vi "STEP SPEED SEQUENCE.vi"(8 "error in (no error)":errorcluster, 11 "main ref":T1) -> (0 "error out":errorcluster)   [LabVIEW 2025]
uses:
  controls/LAB-IQ UI Data.ctl
  Traction Loop/Traction Receipe Enum.ctl
  STEP SPEED SEQUENCE ENUM.ctl
  SWAY vi's/Sway Write enum.ctl
  LOAD CELL CODE/STEP LOAD SEQUENCE ENUM.ctl
panel:
  in  "Checkbox":bool
  out "ELAPSED TIMER":dbl
  out "Test Size":i32
  in  "Time Index":i32
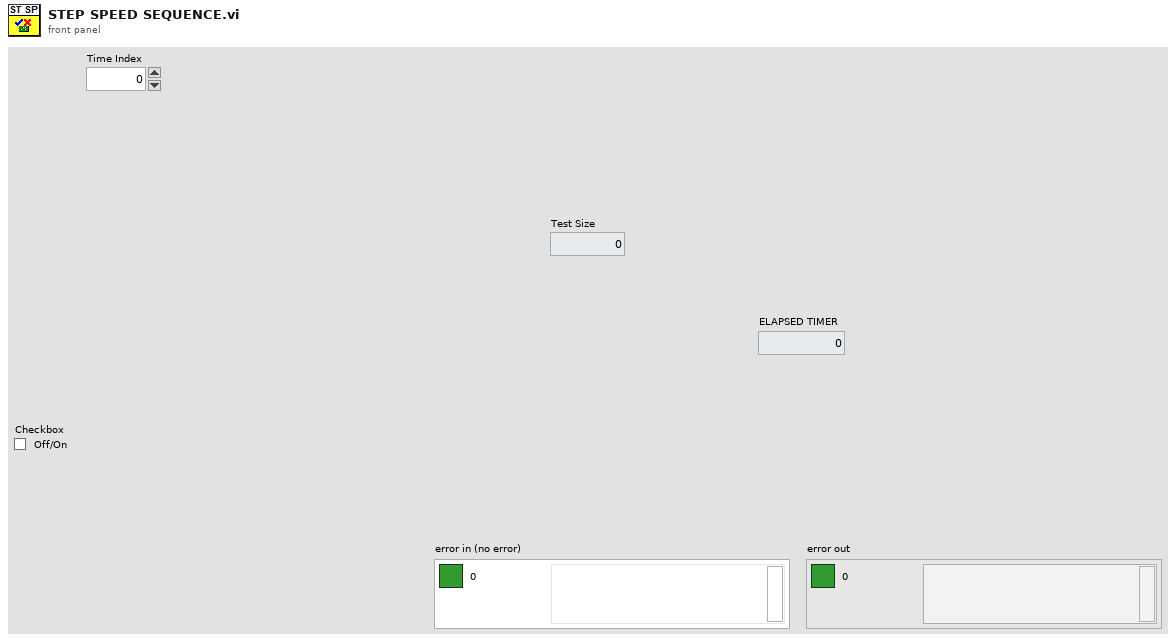
[diagram p1: front panel]
types:
  T1 = typedef "LAB-IQ UI Data.ctl" = cluster{"Main Home Screen":cluster{"GUI":refnum<vi>, "Platform Settings":refnum<vi>, "Configure":refnum<vi>, "Home":refnum<vi>, "EXIT":refnum<vi>, "service 2":refnum<vi>, "MainPage":refnum<vi>, "Analysis":refnum<vi>}, "Platform Settings":cluster{"mm/s  Surge":refnum<vi>, "Drive Error":refnum<vi>, "Disable Axis Jog Soft Limits":refnum<vi>, "mm/s  Sway":refnum<vi>, "Sway and Surge COM Status":refnum<vi>, "Heave COM Status":refnum<vi>, "Enable Platform":refnum<vi>, "Surge Forward Main":refnum<vi>, "Sway Right Main":refnum<vi>, "Sway Left Main":refnum<vi>, "Heave Down Main":refnum<vi>, "Heave Up main":refnum<vi>, "mm/s Heave":refnum<vi>, "mm/sec":refnum<vi>, "mm":refnum<vi>, "Surge Backward Main":refnum<vi>}, "Analysis Screen":cluster{"Analysis Home":refnum<vi>, "Surface Analysis":refnum<vi>, "Imaging":refnum<vi>, "Image Analysis":refnum<vi>, "Post Analysis":refnum<vi>}, "Config Screen":cluster{"Select Load Head":refnum<vi>, "Notes :":refnum<vi>, "FILE":refnum<vi>, "Sample ID :":refnum<vi>, "Operator ID :":refnum<vi>, "Operator Name :":refnum<vi>, "Auto":refnum<vi>}, "Motion Module":cluster{"zNL":refnum<vi>, "NL disp":refnum<vi>, "Rotary Tab":refnum<vi>, "Motion Direction:  3":refnum<vi>, "E.Velocity 2":refnum<vi>, "e.v/ssr 2":refnum<vi>, "Enter Fixed E.Velocity 2":refnum<vi>, "Enter Final SRR 2":refnum<vi>, "Enter initial SRR 2":refnum<vi>, "Enter Fixed SRR 2":refnum<vi>, "Enter the Final E.Velocity (m/s) 2":refnum<vi>, "Enter initial E.Velocity (m/s) 2":refnum<vi>, "Final Speed (RPM) 3":refnum<vi>, "Initial Speed (RPM) 2":refnum<vi>, "Enter the Final Velocity (m/s) 3":refnum<vi>, "Enter initial Velocity (m/s)  3":refnum<vi>, "Ramp Up 2":refnum<vi>, "TEST SELECTION":refnum<vi>, "SPEED SELECTION : ":refnum<vi>, "Angular Oscillation Set":refnum<vi>, "Traction":refnum<vi>, "Step Speed":refnum<vi>, "StepTable For Load-Speed":refnum<vi>, "StepTable For Speed":refnum<vi>, "Surge Forward MM":refnum<vi>, "Surge Backward MM":refnum<vi>, "M3 Image":refnum<vi>, "String 39":refnum<vi>, "Sway Left MM":refnum<vi>, "Sway Right MM":refnum<vi>, "Disable Axis Jog Soft Limits":refnum<vi>, "mm":refnum<vi>, "Heave Down MM":refnum<vi>, "Heave Up MM":refnum<vi>, "Wear Track Diameter (mm)":refnum<vi>, "Set WTD":refnum<vi>, "HomeScratch":refnum<vi>, "HomeRot":refnum<vi>, "PlaceModule":refnum<vi>, "Enter the Angle (Deg)":refnum<vi>, "Enter the Frequency (Hz)":refnum<vi>, "Motion Mode:":refnum<vi>, "LR Sway":refnum<vi>, "Rot Hor":refnum<vi>, "Scratch":refnum<vi>, "LR Cam":refnum<vi>, "MMBack":refnum<vi>, "MMNext":refnum<vi>, "Rot Ver":refnum<vi>, "Rotary Module Selection":refnum<vi>, "calculate rotary":refnum<vi>, "SPEED SELECTION : rotary":refnum<vi>, "Import 2":refnum<vi>, "Save 2":refnum<vi>, "File Path :  2":refnum<vi>, "String 45":refnum<vi>, "StepTable For Speed 3":refnum<vi>, "Enter the Speed(mm/sec)":refnum<vi>, "Enter the Speed(RPM)":refnum<vi>, "Enter Scratch Speed (mm/s):":refnum<vi>, "SwaySpeed Set":refnum<vi>, "Scartch Offset":refnum<vi>, "Motion type:":refnum<vi>, "HomeScratch 2":refnum<vi>, "Enter Scratch length (mm):":refnum<vi>, "Wear Track Diameter":refnum<vi>, "Rotary Speed Exced":refnum<vi>, "Scratch Mode":refnum<vi>, "No of Scratch":refnum<vi>}, "Environmental control":cluster{"Humidity  Status  3":refnum<vi>, "Low Temp  Status  2":refnum<vi>, "TK4 status 2":refnum<vi>, "Stage Temperature":refnum<vi>, "Sample Temperature":refnum<vi>, "Humidity (Amb)":refnum<vi>, "Clear List":refnum<vi>, "Add to list":refnum<vi>, "Wear":refnum<vi>, "Vibration":refnum<vi>, "Humidity (Chamber)":refnum<vi>, "Temperature (Chamber)":refnum<vi>, "ECR ":refnum<vi>, "Temperature (Amb)":refnum<vi>, "Microphone":refnum<vi>, "Acoustic Emission 3":refnum<vi>, "SNext":refnum<vi>, "APBack":refnum<vi>, "Enter the Temperature (°C):":refnum<vi>, "Enter the Stage \nTemperature (°C):":refnum<vi>, "Enter the Humidity (%Rh):":refnum<vi>, "Low Temp":refnum<vi>, "High Temp":refnum<vi>, "Humidity":refnum<vi>, "Sensors Picked":refnum<vi>}, "About Screen":cluster{"Password":refnum<vi>, "Home Service":refnum<vi>, "Advanced Setting":refnum<vi>, "About Tab":refnum<vi>, "ECR Port:":refnum<vi>, "Ramp Port:":refnum<vi>, "Installation/Replacement completed":refnum<vi>, "Loahead":refnum<vi>, "Heave and Surge COM Port:":refnum<vi>, "Sway COM Port:":refnum<vi>, "Temp Modbus:":refnum<vi>, "Humidity Port:":refnum<vi>, "Edit Gain Constants":refnum<vi>, "Save Gain Constants":refnum<vi>}, "Main Screen":cluster{"Main Screen Tab":refnum<vi>, "Angle and Frequency":refnum<vi>, "Stroke (mm)":refnum<vi>, "Angle (Deg)":refnum<vi>, "Main Speed Tab":refnum<vi>, "MTM MOTOR DISPLAY":refnum<vi>, "Disc Speed (m/sec)":refnum<vi>, "Ball Speed (m/sec)":refnum<vi>, "Disc Speed (RPM)":refnum<vi>, "Ball Speed (RPM)":refnum<vi>, "SPEED TAB":refnum<vi>, "Speed (m/sec)":refnum<vi>, "Set Speed (m/sec)":refnum<vi>, "Speed (RPM)":refnum<vi>, "Set Speed":refnum<vi>, "Time Tab":refnum<vi>, "Time ( HH:MM:SS ) 2":refnum<vi>, "Test Duration":refnum<vi>, "Test Duration 4":refnum<vi>, "TEST CYCLE":refnum<vi>, "TOTAL CYCLES":refnum<vi>, "Set Load (N)":refnum<vi>, "Temp Tabs":refnum<vi>, "Heater":refnum<vi>, "TK4 status":refnum<vi>, "ChamberTemp":refnum<vi>, "SetTmp":refnum<vi>, "Controller  Status":refnum<vi>, "ChamberTemp 2":refnum<vi>, "SetTmp 2":refnum<vi>, "Controller  Status 2":refnum<vi>, "ChamberTemp 3":refnum<vi>, "SetTmp 3":refnum<vi>, "Cooling":refnum<vi>, "Load Communication":refnum<vi>, "Ambient \nTemperature":refnum<vi>, "HumCOMStatus":refnum<vi>, "Ambient\n Humidity":refnum<vi>, "Freq (Hz)":refnum<vi>, "Load En":refnum<vi>, "NLt":refnum<vi>, "zNL 2":refnum<vi>, "Humidity On":refnum<vi>, "humidity disp":refnum<vi>, "Set Humidity":refnum<vi>, "NL disp 2":refnum<vi>, "Humidity On 2":refnum<vi>, "humidity disp 2":refnum<vi>, "Set Humidity 2":refnum<vi>, "NL disp 3":refnum<vi>, "AppLoadSeq scratch":refnum<vi>, "Stop Scratch":refnum<vi>, "ClrLog":refnum<vi>, "Trip Log":refnum<vi>, "STOP":refnum<vi>, "Start Test":refnum<vi>, "Test status":refnum<vi>, "AR Led":refnum<vi>, "Data":refnum<vi>, "Health":refnum<vi>, "Sway COM Status":refnum<vi>, "Heave COM Status":refnum<vi>, "Grp Tab":refnum<vi>, "Sub Graph":refnum<vi>, "SD (mm)":refnum<vi>, "Siliding distance Reset Graph":refnum<vi>, "SDGp":refnum<vi>, "Humidity Reset Graph":refnum<vi>, "HumrGp":refnum<vi>, "Acoustic Emission (mV)":refnum<vi>, "Aqucostic Reset Graph":refnum<vi>, "gACQUOS":refnum<vi>, "ECR RESET":refnum<vi>, "ECR":refnum<vi>, "Temperature Reset":refnum<vi>, "Acoustic Emission (mV) 2":refnum<vi>, "Aqucostic Reset Graph 2":refnum<vi>, "gACQUOS 2":refnum<vi>, "ECR RESET 2":refnum<vi>, "ECR 2":refnum<vi>, "Temperature Reset 2":refnum<vi>, "Temperature (deg c)":refnum<vi>, "Speed Reset Graph":refnum<vi>, "Speed Tab":refnum<vi>, "MTM DISC  SPEED":refnum<vi>, "MTM BALL SPEED":refnum<vi>, "speed mm/sec":refnum<vi>, "Hymidity":refnum<vi>, "Humidity Disable trip":refnum<vi>, "CoF Trip  2":refnum<vi>, "Depth Trip":refnum<vi>, "Weart Deapth":refnum<vi>, "Depth Reset Graph":refnum<vi>, "Weart":refnum<vi>, "Depthz":refnum<vi>, "Depth (µm)":refnum<vi>, "WearGp":refnum<vi>, "NL Trip 2":refnum<vi>, "Load pid":refnum<vi>, "Load Disable Trip":refnum<vi>, "Load Reset Graph":refnum<vi>, "NL Display 4":refnum<vi>, "Main Chart 3":refnum<vi>, "BACK":refnum<vi>, "Depth Trip 2":refnum<vi>, "COF TRIP ":refnum<vi>, "Friction Force (N)":refnum<vi>, "FF Reset Graph":refnum<vi>, "FF Disable Trip":refnum<vi>, "FF TRIP":refnum<vi>, "COF Disable Trip":refnum<vi>, "COF Reset Graph":refnum<vi>, "Start Test Temp":refnum<vi>, "zFF":refnum<vi>, "Friction Force (N) Graph":refnum<vi>, "Coefficient of Friction":refnum<vi>, "Scratch Start Test":refnum<vi>, "FF Tab":refnum<vi>, "Cyclic Friction Force (N)":refnum<vi>, "CZ FF":refnum<vi>, "Cyclic Friction Force (N) Graph":refnum<vi>, "Cyclic Coefficient of Friction":refnum<vi>, "Cyclic FF TRIP":refnum<vi>, "Cyclic FF Disable Trip":refnum<vi>, "cyclic COF Disable Trip":refnum<vi>, "cyclic COF TRIP":refnum<vi>, "cyclic COF Reset Graph":refnum<vi>, "Cyclic FF Reset Graph":refnum<vi>, "Test Trip":refnum<vi>, "Multi Scratch Pass":refnum<vi>, "Scratch Start Recording":refnum<vi>}, "Loading":cluster{"Indentation":refnum<vi>, "Reference Sample":refnum<vi>, "Load Cell Communication Slide":refnum<vi>, "com 3":refnum<vi>, "com":refnum<vi>, "DecaForce COM Status":refnum<vi>, "Update":refnum<vi>, "Clear 3":refnum<vi>, "seq":refnum<vi>, "Stribeck table":refnum<vi>, "Stribeck Table  For loading":refnum<vi>, "Loading Mode":refnum<vi>, "Enter the Final Load (N)":refnum<vi>, "Enter the CoF Trip":refnum<vi>, "Enter the Friction Force Trip":refnum<vi>, "Enter the Normal load Trip":refnum<vi>, "Enter the Load  (N)":refnum<vi>, "KiloForce":refnum<vi>, "DecaForce ":refnum<vi>, "MicroForce":refnum<vi>, "LHBack":refnum<vi>, "LHNext":refnum<vi>, "Enter the Loading Rate (N/min)":refnum<vi>, "Message":refnum<vi>, "Warning 2":refnum<vi>, "SSP 0.75":refnum<vi>, "SSP 0.5":refnum<vi>, "SSP 0.3":refnum<vi>, "Warning":refnum<vi>, "gui GIF":refnum<vi>, "Communication is established":refnum<vi>, "AppLoad 4":refnum<vi>, "Multipoint":refnum<vi>, "Load Selection":refnum<vi>}, "PID":cluster{"Ramp":refnum<vi>, "Vertical load (N)":refnum<vi>, "apply load":refnum<vi>, "apply load 2":refnum<vi>, "Enter ByPass Load":refnum<vi>, "Bypass Load":refnum<vi>, "gFF Rot":refnum<vi>}, "Config Parameters":cluster{"Tab Control 3":refnum<vi>, "Tab Control 19":refnum<vi>, "SAMPLES":refnum<vi>, "Re-initilaize":refnum<vi>, "Filter ON/OFF":refnum<vi>, "TracHomeSurgeOffsetCounts 10MM":refnum<vi>, "TracHomeSwayOffsetCounts 10MM":refnum<vi>, "Acoustic Emission:":refnum<vi>, "Apply Filter (FF)":refnum<vi>, "Filter% 2":refnum<vi>, "Apply Filter (Load)":refnum<vi>, "Filter% ":refnum<vi>, "Sway distance (mm)":refnum<vi>, "Surge distance (mm)":refnum<vi>, "DataSavingLoopDelay(ms)":refnum<vi>, "SAVE 2":refnum<vi>, "Enter Distance":refnum<vi>, "Sway Counts:":refnum<vi>, "Distance (mm): 3":refnum<vi>, "Surge Counts:":refnum<vi>, "Distance (mm): 2":refnum<vi>, "Distance (mm):":refnum<vi>, "Heave Counts:":refnum<vi>, "LRMHomeSurgeOffsetCounts":refnum<vi>, "LRMHomeSwayOffsetCounts":refnum<vi>, "TracHomeSurgeOffsetCounts 20MM":refnum<vi>, "TracHomeSwayOffsetCounts 20MM":refnum<vi>, "RotHomeSwayOffsetCounts":refnum<vi>, "RotHomeSurgeOffsetCounts":refnum<vi>, "Heave distance":refnum<vi>, "Zmm":refnum<vi>, "Heave Pulses/mm":refnum<vi>, "Surge Pulses/mm":refnum<vi>, "Sway Pulses/mm":refnum<vi>, "Heave Pitch":refnum<vi>, "Surge Pitch":refnum<vi>, "Sway Pitch":refnum<vi>, "Heave PPR":refnum<vi>, "Surge PPR":refnum<vi>, "Sway PPR":refnum<vi>, "Tab Control 5":refnum<vi>, "Tab Control 14":refnum<vi>, "Tab Control 26":refnum<vi>, "AE":refnum<vi>, "Heave Loop Delay":refnum<vi>, "Heave PID Speed":refnum<vi>, "Surge Jog Speed":refnum<vi>, "Heave Jog Speed":refnum<vi>, "Sway Loop Delay":refnum<vi>, "Sway PID Speed":refnum<vi>, "Sway Jog Speed":refnum<vi>, "DEPTH TRIP VALUE":refnum<vi>, "LOAD TRIP VALUE":refnum<vi>, "DEPTH TRIP   ENABLE":refnum<vi>, "LOAD TRIP  ENABLE":refnum<vi>, "CYCLIC FF TRIP VALUE":refnum<vi>, "FF TRIP VALUE":refnum<vi>, "CYCLIC CoF TRIP VALUE":refnum<vi>, "COF TRIP VALUE":refnum<vi>, "CYCLIC COF TRIP  ENABLE":refnum<vi>, "CYCLIC FF TRIP  ENABLE":refnum<vi>, "FF TRIP  ENABLE":refnum<vi>, "COF TRIP  ENABLE":refnum<vi>, "JOG TRIP LOAD VALUE (N)":refnum<vi>, "Rotary Vertical":refnum<vi>, "Traction":refnum<vi>, "Scratch":refnum<vi>, "LRM CAM":refnum<vi>, "Sway LRM":refnum<vi>, "Rotary Horizontal":refnum<vi>}, "Loading Com Port":cluster{"ClearAll":refnum<vi>, "Mz(Nm)":refnum<vi>, "My(Nm)":refnum<vi>, "Mx(Nm)":refnum<vi>, "Save Dwell":refnum<vi>, "Acq Delay (ms)":refnum<vi>, "Burst Delay (ms)":refnum<vi>, "model":refnum<vi>, "SN":refnum<vi>, "FFx(N)":refnum<vi>, "Sensor IP":refnum<vi>, "Port":refnum<vi>, "FFy(N)":refnum<vi>, "Load(N)":refnum<vi>, "delete Handle":refnum<vi>, "Create Handle":refnum<vi>, "ft_data":refnum<vi>, "ft_range":refnum<vi>, "ft_data 2":refnum<vi>, "stop 6":refnum<vi>, "running_flag":refnum<vi>, "ft_udp_handle":refnum<vi>, "get-data-return":refnum<vi>, "get-range-return":refnum<vi>, "zero-return":refnum<vi>, "filter-return":refnum<vi>, "initial-return":refnum<vi>, "deleteHandle-result":refnum<vi>, "Load Cell Temp":refnum<vi>, "Load Cell":refnum<vi>, "ZeroAll":refnum<vi>, "FORCE (N)":refnum<vi>, "TORQUE (N-m)":refnum<vi>, "Load Cell Link":refnum<vi>}, "Heave AND Surge":cluster{"SURGE POSE":refnum<vi>, "error out Read":refnum<vi>, "HEAVE POSE":refnum<vi>, "State":refnum<vi>, "Homed":refnum<vi>, "Sequence ID":refnum<vi>, "error out Write":refnum<vi>, "faultCode":refnum<vi>, "Ack ID":refnum<vi>, "SPEED":refnum<vi>, "Distance":refnum<vi>, "Mode Command":refnum<vi>, "Heave and Surge Read":refnum<vi>, "Read Heave Temp":refnum<vi>, "Spare 15":refnum<vi>, "Spare 14":refnum<vi>, "Spare 13":refnum<vi>, "Spare 12":refnum<vi>, "Spare 11":refnum<vi>, "Spare 10":refnum<vi>, "Spare 9":refnum<vi>, "Spare 8":refnum<vi>, "Spare 7":refnum<vi>, "Spare 4":refnum<vi>, "Spare 3":refnum<vi>, "Spare 2":refnum<vi>, "Humidity":refnum<vi>, "Temp":refnum<vi>, "Node Id":refnum<vi>, "Spare 1":refnum<vi>, "SPARE 4":refnum<vi>, "SPARE 3":refnum<vi>, "SPARE 2":refnum<vi>, "SPARE 1":refnum<vi>, "fwMajor":refnum<vi>, "fwMinor":refnum<vi>, "Manual Write":refnum<vi>, "Heave and Surge Write":refnum<vi>, "SPARE 5":refnum<vi>, "Reserved ":refnum<vi>, "SPARE 8":refnum<vi>, "SPARE 6":refnum<vi>, "SPARE 7":refnum<vi>, "SPARE 17":refnum<vi>, "SPARE 16":refnum<vi>, "SPARE 15":refnum<vi>, "SPARE 14":refnum<vi>, "SPARE 13":refnum<vi>, "SPARE 12":refnum<vi>, "SPARE 11":refnum<vi>, "SPARE 10":refnum<vi>, "SPARE 9":refnum<vi>, "System UPTIME":refnum<vi>, "Missed Packets":refnum<vi>, "faultCode Surge Right":refnum<vi>, "faultCode Surge Left":refnum<vi>, "faultCode Heave":refnum<vi>, "UPLINK HEAVE":refnum<vi>, "DOWNLINK HEAVE":refnum<vi>}, "New PID LOGIC":cluster{"Fine Tune Zone":refnum<vi>, "PID SDelay":refnum<vi>, "Max_pos_limit":refnum<vi>, "Min_pos_limit":refnum<vi>, "i_limit":refnum<vi>, "pct_scale":refnum<vi>, "Deadband":refnum<vi>, "Kd":refnum<vi>, "Ki":refnum<vi>, "Kp":refnum<vi>, "Current Position":refnum<vi>, "Set Load":refnum<vi>, "Current Load":refnum<vi>, "Pulse delta":refnum<vi>, "Init Step":refnum<vi>, "Max Step Linit":refnum<vi>, "min_deadband_floor":refnum<vi>, "dynamic_spindle_noise_scalar":refnum<vi>, "min_finetune_floor":refnum<vi>, "filter_alpha":refnum<vi>, "PID":refnum<vi>}, "SWAY ":cluster{"fwMajor":refnum<vi>, "Homed":refnum<vi>, "Rotary POSE":refnum<vi>, "State":refnum<vi>, "SWAY POSE":refnum<vi>, "Ack ID":refnum<vi>, "faultCode":refnum<vi>, "Node Id":refnum<vi>, "fwMinor":refnum<vi>, "Spare 6":refnum<vi>, "Spare 5":refnum<vi>, "Spare 4":refnum<vi>, "Spare 3":refnum<vi>, "Spare 2":refnum<vi>, "Spare 1":refnum<vi>, "Spare 7":refnum<vi>, "SPARE  5":refnum<vi>, "error out Write  SWAY ":refnum<vi>, "error out Read SWAY ":refnum<vi>, "Manual Write SWAY ":refnum<vi>, "SWAY WRITE":refnum<vi>, "SPARE  4":refnum<vi>, "SPARE  3":refnum<vi>, "SPARE 2":refnum<vi>, "SPARE 1":refnum<vi>, "Spare 15":refnum<vi>, "Spare 14":refnum<vi>, "Spare 13":refnum<vi>, "Spare 12":refnum<vi>, "Spare 11":refnum<vi>, "Spare 9":refnum<vi>, "Spare 8":refnum<vi>, "SPEED":refnum<vi>, "Distance":refnum<vi>, "Mode Command":refnum<vi>, "Sequence ID":refnum<vi>, "SWAY READ":refnum<vi>, "Spare 10":refnum<vi>, "Read SWAY Temp":refnum<vi>, "faultCode Sway ":refnum<vi>, "Missed Packets":refnum<vi>, "System UPTIME sway":refnum<vi>, "SPARE 6":refnum<vi>, "SPARE 7":refnum<vi>, "SPARE 9":refnum<vi>, "SPARE 11":refnum<vi>, "SPARE 10":refnum<vi>, "SPARE 8":refnum<vi>, "SPARE 13":refnum<vi>, "SPARE 12":refnum<vi>, "SPARE 17":refnum<vi>, "SPARE 16":refnum<vi>, "SPARE 15":refnum<vi>, "SPARE 14":refnum<vi>, "Reserved":refnum<vi>, "faultCode Rotary":refnum<vi>, "UPLINK SWAY":refnum<vi>, "DOWNLINK SWAY":refnum<vi>}, "Analysis Screen":cluster{"Analysis Home":refnum<vi>, "Refresh 2":refnum<vi>, "MEAN 4":refnum<vi>, "SD 4":refnum<vi>, "VARIANCE 4":refnum<vi>, "MEAN  3":refnum<vi>, "SD  3":refnum<vi>, "VARIANCE  3":refnum<vi>, "MEAN 2":refnum<vi>, "SD  2":refnum<vi>, "VARIANCE 2":refnum<vi>, "MEAN":refnum<vi>, "SD":refnum<vi>, "VARIANCE":refnum<vi>, "File 4 Discription":refnum<vi>, "OPEN 4":refnum<vi>, "File Name 4":refnum<vi>, "OPEN 3":refnum<vi>, "File 3 Discription":refnum<vi>, "File Name 3":refnum<vi>, "Y-AXIS":refnum<vi>, "X-AXIS":refnum<vi>, "XY Graph":refnum<vi>, "File Name 2":refnum<vi>, "File Name 1":refnum<vi>, "OPEN 2":refnum<vi>, "OPEN 1":refnum<vi>, "File 1 Discription ":refnum<vi>, "File 2 Discription":refnum<vi>, "Export":refnum<vi>, "File Format":refnum<vi>}, "Traction":cluster{"faultCode Traction 2":refnum<vi>, "faultCode Traction 1":refnum<vi>, "Missed Packets":refnum<vi>, "System UPTIME Traction":refnum<vi>, "SPARE 17":refnum<vi>, "SPARE 16":refnum<vi>, "SPARE 15":refnum<vi>, "SPARE 14":refnum<vi>, "SPARE 13":refnum<vi>, "SPARE 12":refnum<vi>, "SPARE 11":refnum<vi>, "SPARE 10":refnum<vi>, "SPARE 9":refnum<vi>, "SPARE 8":refnum<vi>, "SPARE 7":refnum<vi>, "SPARE 6":refnum<vi>, "Reserved":refnum<vi>, "SPARE  5":refnum<vi>, "Manual Write TRACTION":refnum<vi>, "TRACTION WRITE":refnum<vi>, "SPARE  4":refnum<vi>, "SPARE  3":refnum<vi>, "SPARE 2":refnum<vi>, "SPARE 1":refnum<vi>, "Spare 7":refnum<vi>, "Spare 6":refnum<vi>, "Spare 5":refnum<vi>, "Spare 4":refnum<vi>, "Spare 2":refnum<vi>, "Spare 1":refnum<vi>, "Node Id":refnum<vi>, "Read TRACTION Temp":refnum<vi>, "fwMinor":refnum<vi>, "fwMajor":refnum<vi>, "faultCode":refnum<vi>, "TRACTION POSE":refnum<vi>, "TRACTION POSE 2":refnum<vi>, "Homed":refnum<vi>, "State":refnum<vi>, "Ack ID":refnum<vi>, "SPEED":refnum<vi>, "Distance":refnum<vi>, "Mode Command":refnum<vi>, "Sequence ID":refnum<vi>, "error out Read TRACTION":refnum<vi>, "error out Write  TRACTION":refnum<vi>, "TRACTION READ":refnum<vi>, "Spare 3":refnum<vi>, "Downlink traction":refnum<vi>, "Uplink Traction":refnum<vi>}, "Traction reciepe":cluster{"SRR Sweep Range (%) Stribeck":refnum<vi>, "Traction Receipe":refnum<vi>, "Total Execution Time":refnum<vi>, "Total Steps":refnum<vi>, "Duration / Step (s)  Stribeck":refnum<vi>, "STRIBECK Fixed SRR List (%)":refnum<vi>, "Duration / Step (s) Traction":refnum<vi>, "SRR Sweep Range (%) traction":refnum<vi>, "Rolling Speed (mm/s)":refnum<vi>, "Temperature Stages (°C)":refnum<vi>, "Ball Load (N)":refnum<vi>, "Lubricant Name":refnum<vi>, "Profile File Name":refnum<vi>, "SET entrainment Velocity":refnum<vi>, "Test Array Size":refnum<vi>, "SRR INDEX [ STRIBECK]":refnum<vi>, "Stribeck Size":refnum<vi>, "SET SRR":refnum<vi>, "ELAPSED TIMER ":refnum<vi>, "BALL SET RPM":refnum<vi>, "DISC SET RPM":refnum<vi>, "SET LOAD":refnum<vi>, "TEMPERATURE READ":refnum<vi>, "SET TEMPERATURE":refnum<vi>, "Traction Size":refnum<vi>, "DISC SPEED (rpm)":refnum<vi>, "BALL SPEED (rpm)":refnum<vi>, "BALL WEAR TRACK":refnum<vi>, "DISC WEARTRACK":refnum<vi>, "SRR INDEX [ TRACTION]":refnum<vi>, "Start Index Type":refnum<vi>, "Enum - Menu":refnum<vi>, "Ball (mm/sec)":refnum<vi>, "Disc (mm/sec)":refnum<vi>}, "Traction Control":cluster{"HomeTraction":refnum<vi>, "Demo Mode Display":refnum<vi>, "Traction Message":refnum<vi>, "Traction Step Update Details":refnum<vi>, "Main Tab sequence for selection":refnum<vi>, "Ramp Tab":refnum<vi>, "e.v/ssr":refnum<vi>, "Enter Fixed E.Velocity":refnum<vi>, "Enter Final SRR":refnum<vi>, "Enter initial SRR":refnum<vi>, "Enter Fixed SRR":refnum<vi>, "Enter the Final E.Velocity (m/s)":refnum<vi>, "Enter initial E.Velocity (m/s)":refnum<vi>, "Ball WTD":refnum<vi>, "E.Velocity":refnum<vi>, "Enter the Final Velocity (m/s)":refnum<vi>, "Enter initial Velocity (m/s)":refnum<vi>, "Ramp Up   Disc":refnum<vi>, "Initial DiscSpeed (RPM)":refnum<vi>, "Final Speed (RPM) Ball":refnum<vi>, "Final Speed (RPM)":refnum<vi>, "Initial Speed (RPM) Ball":refnum<vi>, "Enter the Final Velocity (m/s) Ball":refnum<vi>, "Enter initial Velocity (m/s) Ball":refnum<vi>, "Ramp Up":refnum<vi>, "ExceedBallSpeed step":refnum<vi>, "ExceedDiscSpeed":refnum<vi>, "BallSpeed Exceed Indication":refnum<vi>, "Apply":refnum<vi>, "SPEED SELECTION : MTM":refnum<vi>, "SPEED SELECTION : MTM 2":refnum<vi>, "TEST SELECTION (MTM)":refnum<vi>, "MTM Test Selection":refnum<vi>, "File Path Tab":refnum<vi>, "File Path String":refnum<vi>, "Save":refnum<vi>, "Save  2":refnum<vi>, "Import ":refnum<vi>, "File Path :":refnum<vi>, "Step Sequence Indication Tab":refnum<vi>, "Step Sequence Indication":refnum<vi>, "Calculate Step":refnum<vi>, "StepTable":refnum<vi>, "ExceedDiscSpeed  Cinstant Speed":refnum<vi>, "ExceedBallSpeed Constant":refnum<vi>, "TEST SELECTION (MTM) 2":refnum<vi>, "SPEED SELECTION : MTM 3":refnum<vi>, "MTM Test Selection 2":refnum<vi>, "Enter the Speed (m/sec): ":refnum<vi>, "Enter the Speed (m/sec):  2":refnum<vi>, "Enter the Speed (RPM):":refnum<vi>, "Lower Spped ":refnum<vi>, "Upper":refnum<vi>, "Enter the Speed (RPM):Ball":refnum<vi>, "Disc Motion Direction: ":refnum<vi>, "Ball Motion Direction :":refnum<vi>, "Motion Mode: ":refnum<vi>, "Wear Track Diameter (mm) ":refnum<vi>, "Disc Speed Indicator":refnum<vi>, "ExceedBallSpeed":refnum<vi>}, "Acquostic":cluster{"Last Config Rejected ":refnum<vi>, "rx command count":refnum<vi>, "Current Filter Id":refnum<vi>, "Isolated Gain":refnum<vi>, "DAQ Status":refnum<vi>, "error out":refnum<vi>, "error in (no error)":refnum<vi>, "Uplink Packet":refnum<vi>, "data out":refnum<vi>, "Downlink Packet":refnum<vi>, "Gains":refnum<vi>, "Manual Write Acquostic":refnum<vi>, "Acoustic Graphs":refnum<vi>}}
  T2 = enum32{"Setup", "Load Head", "Motion Module", "Environment", "Begin"}
  T3 = typedef "STEP SPEED SEQUENCE ENUM.ctl" = enum16{"INIT", "TEST START", "TEST INCREMENT", "TEST STOP"}
  T4 = cluster{"Sequence ID":u16, "Mode Command":u8, "Distance":sgl, "SPEED":sgl, "Reserved":sgl, "SPARE 1":u8, "SPARE 2":u8, "SPARE 3":u8, "SPARE 4":u8, "SPARE 5":u8, "SPARE 6":u8, "SPARE 7":u8, "SPARE 8":u8, "SPARE 9":u8, "SPARE 10":u8, "SPARE 11":u8, "SPARE 12":u8, "SPARE 13":u8, "SPARE 14":u8, "SPARE 15":u8, "SPARE 16":u8, "SPARE 17":u8}
  T5 = typedef "Sway Write enum.ctl" = enum16{"INIT", "WRITE", "CLOSE", "REINIT"}
  T6 = typedef "STEP LOAD SEQUENCE ENUM.ctl" = enum16{"INIT", "TEST START", "TEST INCREMENT", "TEST STOP"}
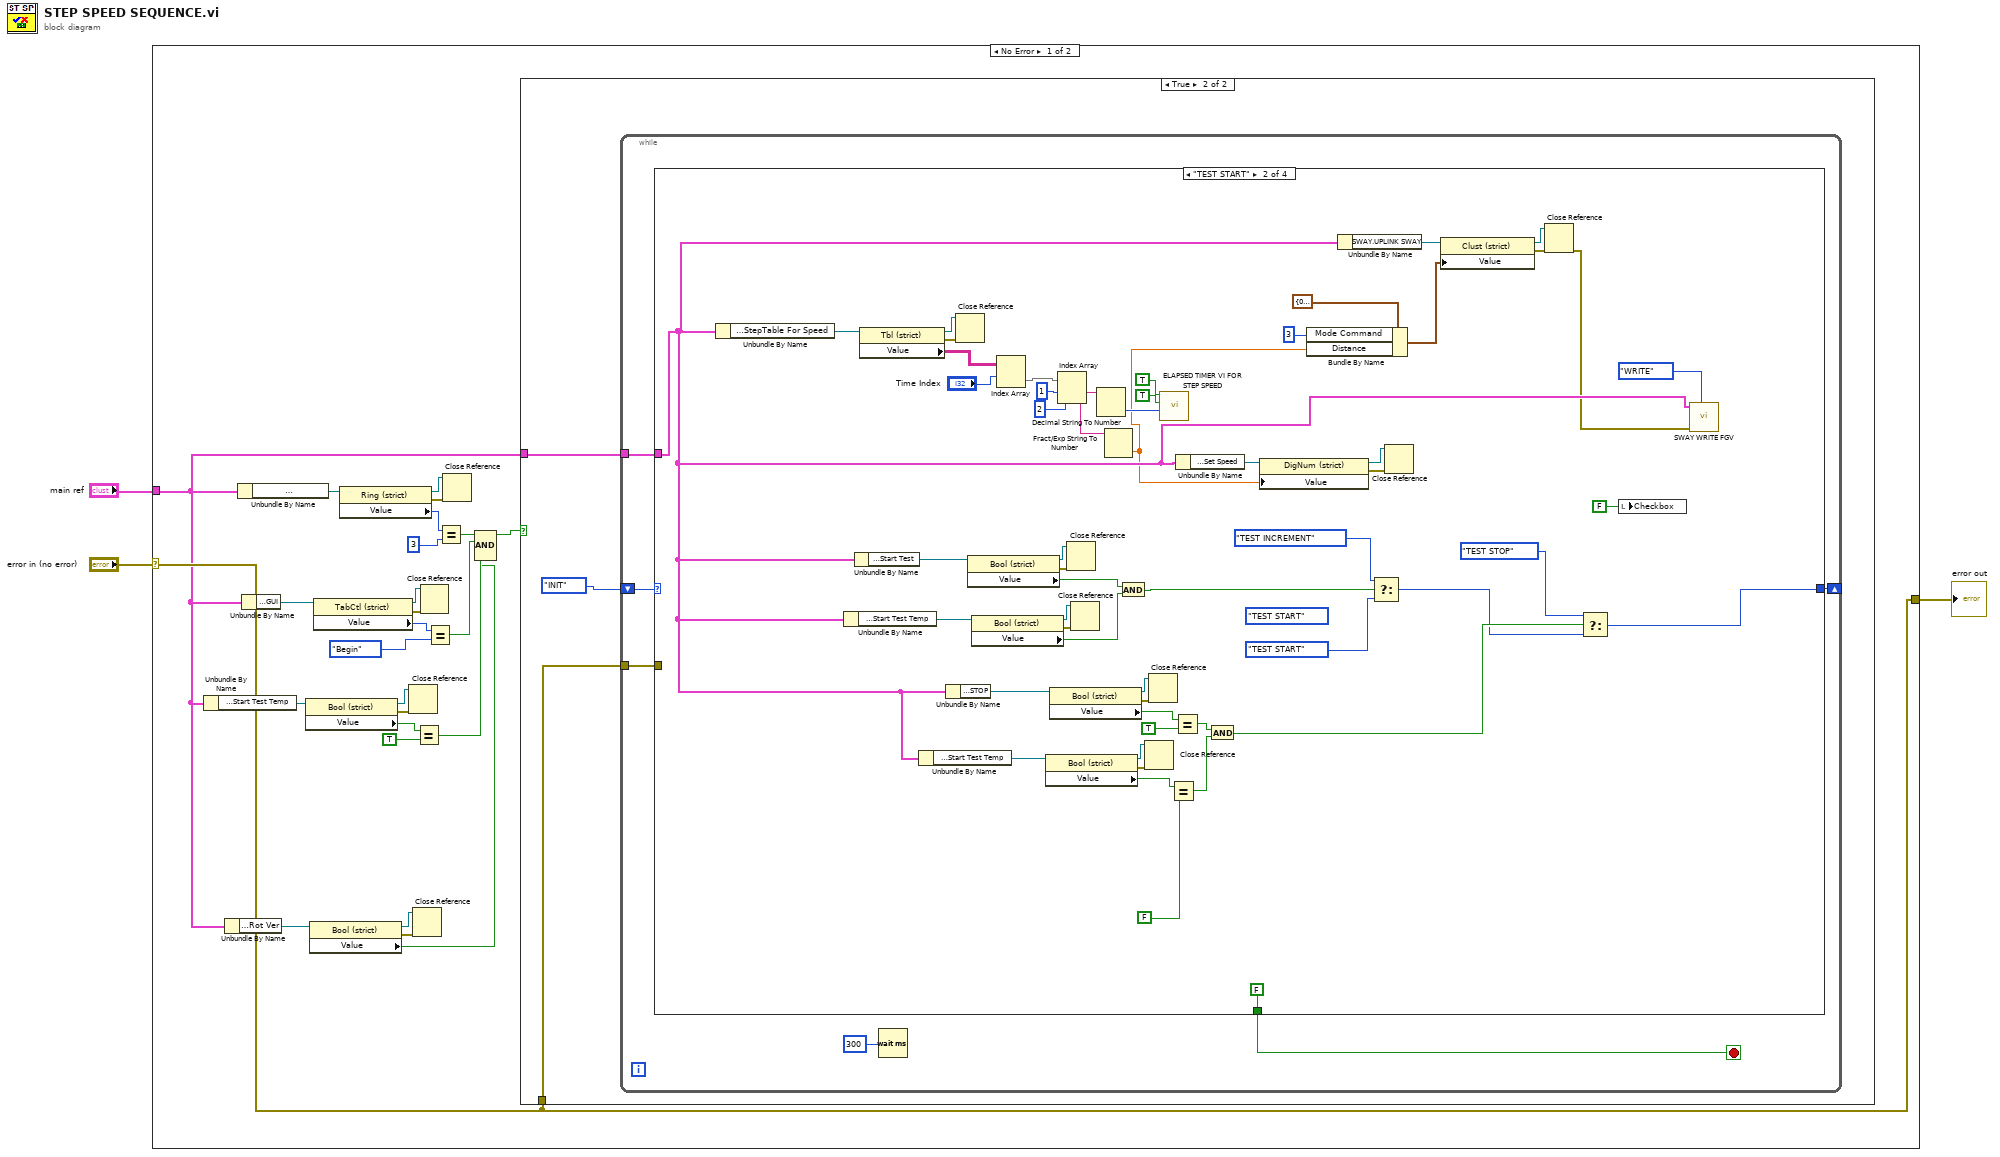
[diagram p0: block diagram]
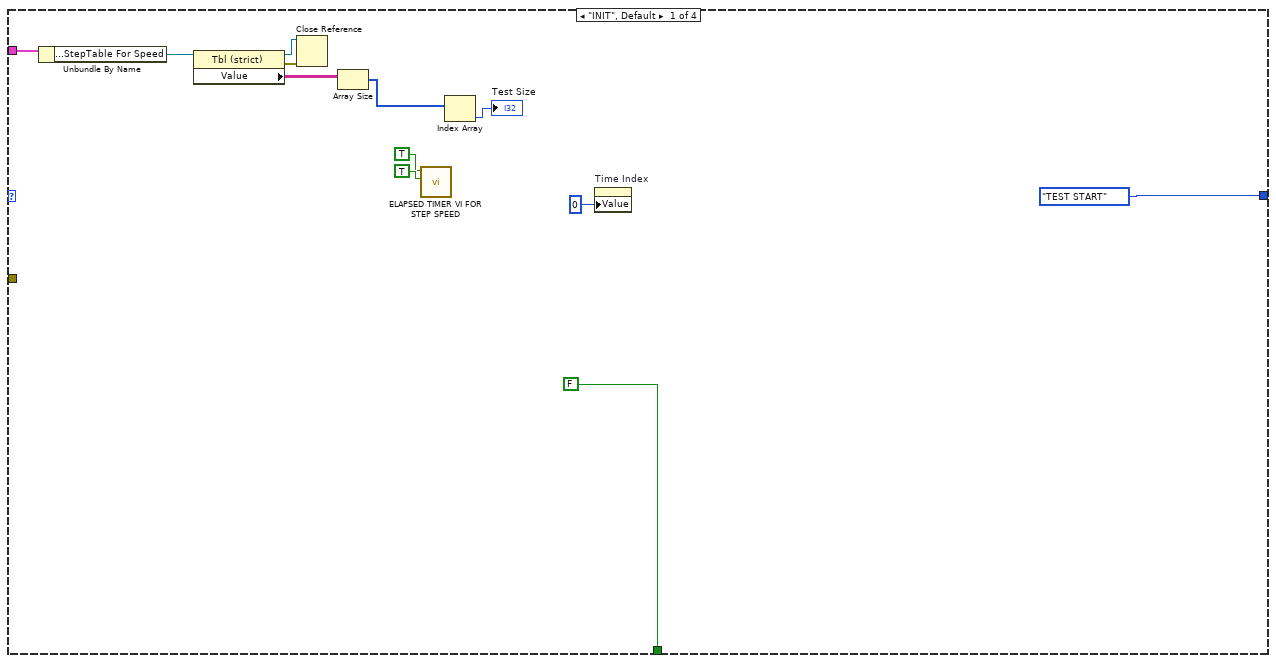
[diagram p3: hidden frame]
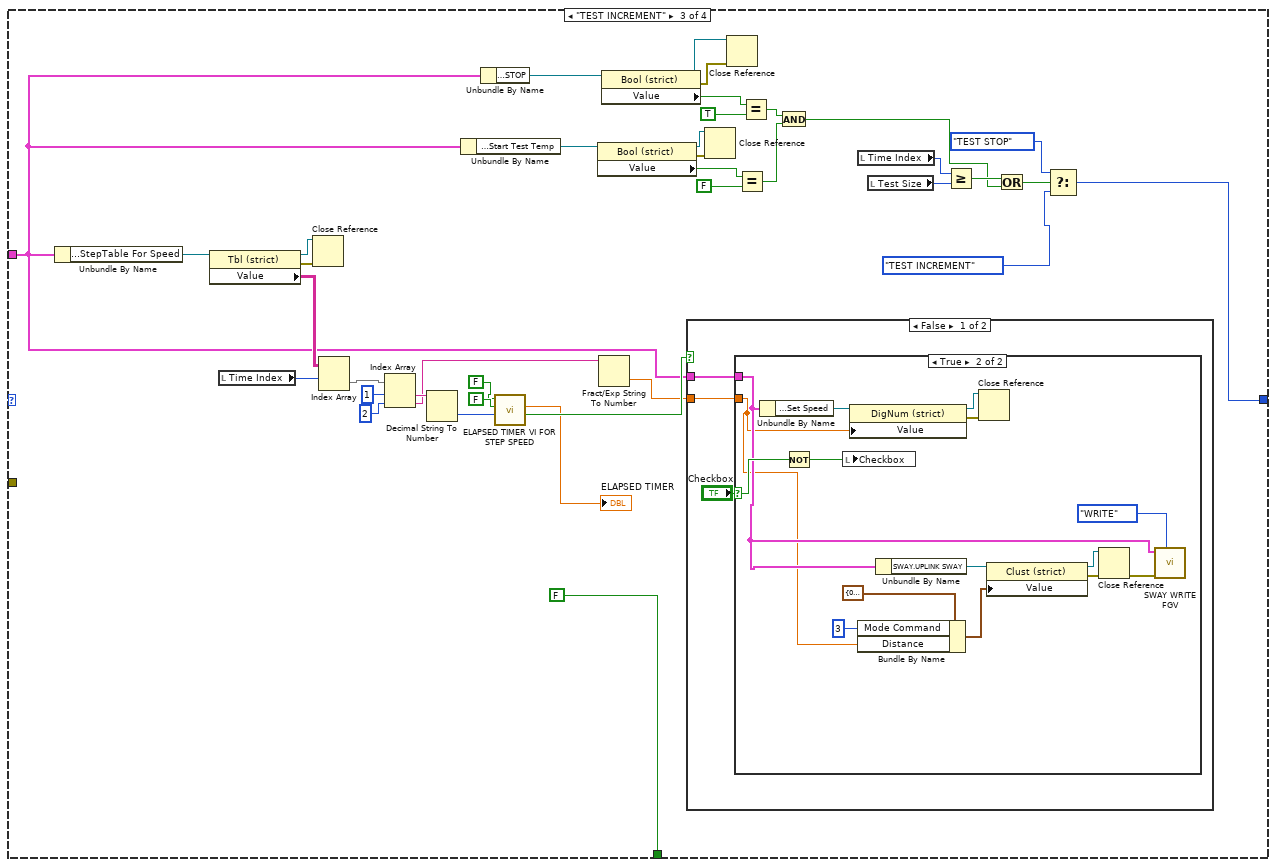
[diagram p4: hidden frame]
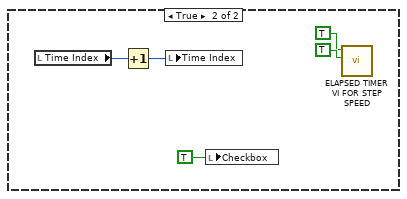
[diagram p6: hidden frame]
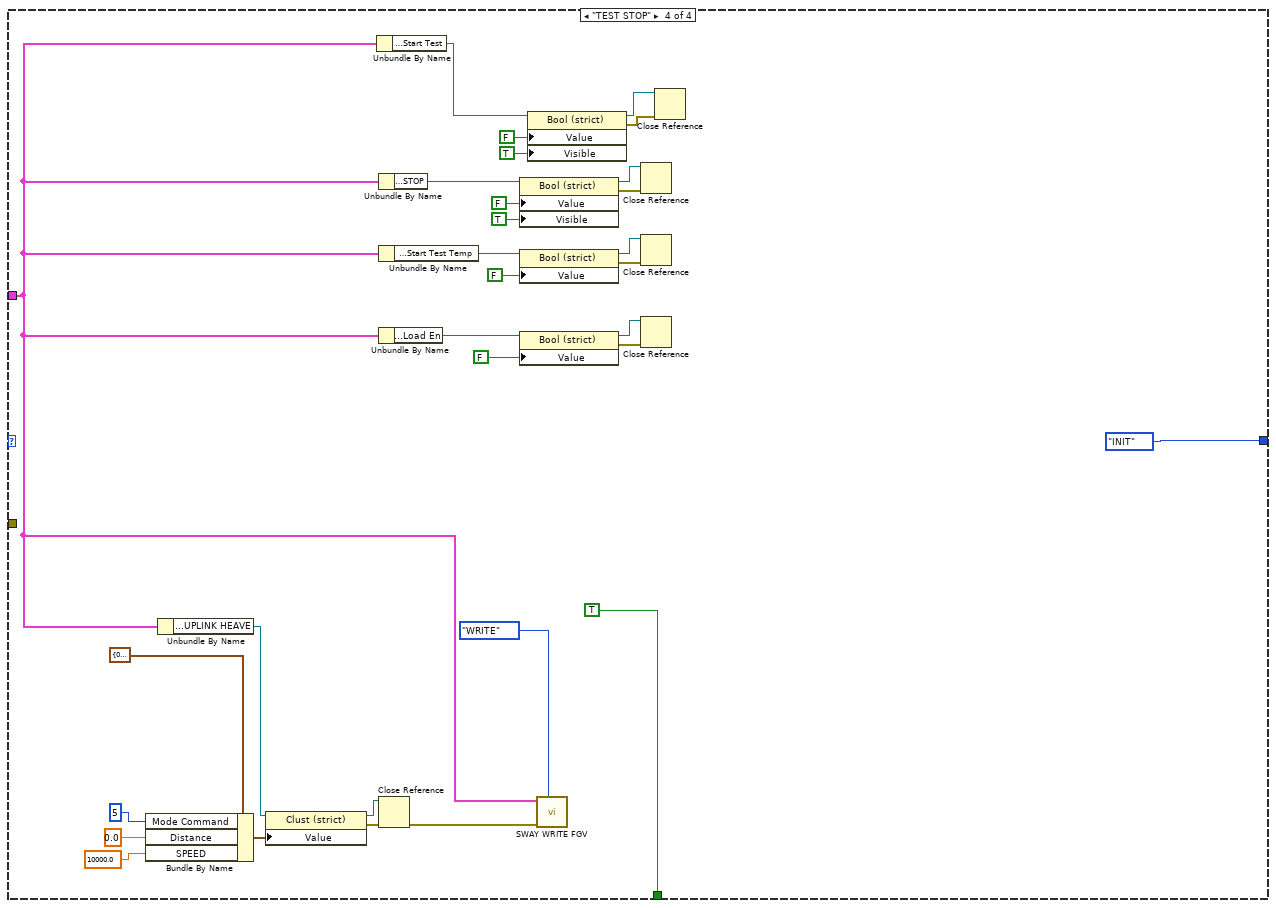
[diagram p7: hidden frame]
diagram:
  n1 = case shown="No Error" "error in (no error)" {
    selector: "error in (no error)" -> [w9 _]
    tunnel: "main ref" -> [w6 _]
    tunnel: [w9 _] -> w1
    frame No Error {
      n2 = Unbundle By Name(w6) -> ("Main Screen.Start Test Temp"=w14:refnum<vi>)
      n3 = Unbundle By Name(w6) -> ("Motion Module.Rot Ver"=w8:refnum<vi>)
      n4 = Unbundle By Name(w6) -> ("Motion Module.Motion Mode:"=w28:refnum<vi>)
      n5 = Unbundle By Name(w6) -> ("Main Home Screen.GUI"=w20:refnum<vi>)
      n6 = property class="Bool (strict)"(reference=w14) -> (reference out=w12:refnum<vi>, error out=w13:errorcluster, "Value"=w15:bool)  [unwired: 1 in]
      n7 = property class="Bool (strict)"(reference=w8) -> (reference out=w4:refnum<vi>, error out=w7:errorcluster, "Value"=w5:bool)  [unwired: 1 in]
      n8 = property class="TabCtl (strict)"(reference=w20) -> (reference out=w22:refnum<vi>, error out=w21:errorcluster, "Value"=w18:T2)  [unwired: 1 in]
      n9 = property class="Ring (strict)"(reference=w28) -> (reference out=w26:refnum<vi>, error out=w27:errorcluster, "Value"=w25:u16)  [unwired: 1 in]
      n10 = Close Reference(reference=w12, error in (no error)=w13) -> ()  [unwired: 1 out]
      n11 = Close Reference(reference=w4, error in (no error)=w7) -> ()  [unwired: 1 out]
      n12 = Equal?(x=w15, y=TRUE) -> (x = y?=w11:bool)
      n13 = Close Reference(reference=w22, error in (no error)=w21) -> ()  [unwired: 1 out]
      n14 = Equal?(x=w18, y=T2."Begin" ("Value")) -> (x = y?=w16:bool)
      n15 = Equal?(x=w25, y=u16 3 ("Value")) -> (x = y?=w23:bool)
      n16 = Close Reference(reference=w26, error in (no error)=w27) -> ()  [unwired: 1 out]
      n17 = Compound Arithmetic op=AND(w23, w16, w11, w5) -> (w19:bool)
      n18 = case shown="True" w19 {
        tunnel: w6 -> [_ w30]
        tunnel: w9 -> [_ w29]
        frame False {
        }
        frame True {
          n19 = while {
            shift-right: [w36] -> _
            shift-left: STEP_SPEED_SEQUENCE_ENUM."INIT" -> [w37]
            tunnel: w30 -> [w34]
            tunnel: w29 -> [w33]
            stop <- w35 stop-if-true
            n20 = case shown="\"TEST START\"" w37 {
              tunnel: [STEP_SPEED_SEQUENCE_ENUM."TEST START" w69 w127 STEP_SPEED_SEQUENCE_ENUM."INIT"] -> w36
              tunnel: [FALSE FALSE FALSE TRUE] -> w35
              tunnel: w34 -> [w40 w52 w107 w166]
              tunnel: w33 -> [_ _ _ _]
              frame "INIT", Default {
                n21 = Unbundle By Name(w40) -> ("Motion Module.StepTable For Speed"=w43:refnum<vi>)
                n22 = property class="Tbl (strict)"(reference=w43) -> (reference out=w41:refnum<vi>, error out=w42:errorcluster, "Value"=w39:string[][])  [unwired: 1 in]
                n23 = Close Reference(reference=w41, error in (no error)=w42) -> ()  [unwired: 1 out]
                n24 = Array Size(array=w39) -> (size(s)=w46:i32[])
                n25 = call "ELAPSED TIMER VI FOR STEP SPEED.vi"("RESET"=TRUE, "PAUSE"=TRUE) -> ()  [unwired: 7 in, 3 out]
                n26 = Index Array(array=w46) -> (element=→"Test Size":i32)  [unwired: 1 in]
                n27 = property on="Time Index" class="DigNum (strict)"("Value"=0 ("Time Index")) -> ()  [unwired: 2 in, 2 out]
              }
              frame "TEST START" {
                (unwired) STEP_LOAD_SEQUENCE_ENUM."TEST START"
                n28 = Unbundle By Name(w52) -> ("Motion Module.StepTable For Speed"=w97:refnum<vi>)
                n29 = Unbundle By Name(w52) -> ("Main Screen.Start Test Temp"=w90:refnum<vi>)
                n30 = Unbundle By Name(w52) -> ("Main Screen.Start Test"=w91:refnum<vi>)
                n31 = property class="Tbl (strict)"(reference=w97) -> (reference out=w95:refnum<vi>, error out=w96:errorcluster, "Value"=w94:string[][])  [unwired: 1 in]
                n32 = Unbundle By Name(w52) -> ("Main Screen.Start Test Temp"=w77:refnum<vi>)
                n33 = Unbundle By Name(w52) -> ("Main Screen.STOP"=w82:refnum<vi>)
                n34 = Close Reference(reference=w95, error in (no error)=w96) -> ()  [unwired: 1 out]
                n35 = property class="Bool (strict)"(reference=w91) -> (reference out=w93:refnum<vi>, error out=w92:errorcluster, "Value"=w87:bool)  [unwired: 1 in]
                n36 = property class="Bool (strict)"(reference=w90) -> (reference out=w88:refnum<vi>, error out=w89:errorcluster, "Value"=w86:bool)  [unwired: 1 in]
                n37 = Index Array(array=w94, index (row)="Time Index") -> (element=w103:string[])  [unwired: 1 in]
                n38 = property class="Bool (strict)"(reference=w77) -> (reference out=w75:refnum<vi>, error out=w76:errorcluster, "Value"=w78:bool)  [unwired: 1 in]
                n39 = property class="Bool (strict)"(reference=w82) -> (reference out=w84:refnum<vi>, error out=w83:errorcluster, "Value"=w81:bool)  [unwired: 1 in]
                n40 = Index Array(array=w103, index #1=1 ("index"), index #2=2 ("index")) -> (element #1=w101:string, element #2=w64:string)
                n41 = Close Reference(reference=w93, error in (no error)=w92) -> ()  [unwired: 1 out]
                n42 = Close Reference(reference=w88, error in (no error)=w89) -> ()  [unwired: 1 out]
                n43 = Decimal String To Number(string=w101) -> (number=w98:i32)  [unwired: 2 in, 1 out]
                n44 = Fract/Exp String To Number(string=w64) -> (number=w51:dbl)  [unwired: 3 in, 1 out]
                n45 = And(x=w87, y=w86) -> (x .and. y?=w85:bool)
                n46 = Close Reference(reference=w75, error in (no error)=w76) -> ()  [unwired: 1 out]
                n47 = Close Reference(reference=w84, error in (no error)=w83) -> ()  [unwired: 1 out]
                n48 = call "ELAPSED TIMER VI FOR STEP SPEED.vi"("TARGET"=w98, "RESET"=TRUE, "PAUSE"=TRUE) -> ()  [unwired: 6 in, 3 out]
                n49 = Equal?(x=w78, y=FALSE) -> (x = y?=w73:bool)
                n50 = Equal?(x=w81, y=TRUE) -> (x = y?=w74:bool)
                n51 = Unbundle By Name(w52) -> ("Main Screen.Set Speed"=w63:refnum<vi>)
                n52 = And(x=w74, y=w73) -> (x .and. y?=w71:bool)
                n53 = property class="DigNum (strict)"(reference=w63, "Value"=w51) -> (reference out=w61:refnum<vi>, error out=w62:errorcluster)  [unwired: 1 in]
                n54 = Bundle By Name(cluster=T4 {"Sequence ID"=0, "Mode Command"=0, "Distance"=0.0, "SPEED"=0.0, "Reserved"=0.0, "SPARE 1"=0, "SPARE 2"=0, "SPARE 3"=0, "SPARE 4"=0, "SPARE 5"=0, "SPARE 6"=0, "SPARE 7"=0, "SPARE 8"=0, "SPARE 9"=0, "SPARE 10"=0, "SPARE 11"=0, "SPARE 12"=0, "SPARE 13"=0, "SPARE 14"=0, "SPARE 15"=0, "SPARE 16"=0, "SPARE 17"=0} ("Value"), "Mode Command"=u8 3, "Distance"=w51) -> (w54:T4)
                n55 = Unbundle By Name(w52) -> ("SWAY.UPLINK SWAY"=w56:refnum<vi>)
                n56 = Select(t=STEP_SPEED_SEQUENCE_ENUM."TEST INCREMENT", s=w85, f=STEP_SPEED_SEQUENCE_ENUM."TEST START") -> (s? t:f=w70:T3)
                n57 = Close Reference(reference=w61, error in (no error)=w62) -> ()  [unwired: 1 out]
                n58 = property on="Property Node" class="Clust (strict)"(reference=w56, "Value"=w54) -> (reference out=w58:refnum<vi>, error out=w57:errorcluster)  [unwired: 1 in]
                n59 = Close Reference(reference=w58, error in (no error)=w57) -> (error out=w50:errorcluster)
                n60 = Select(t=STEP_SPEED_SEQUENCE_ENUM."TEST STOP", s=w71, f=w70) -> (s? t:f=w69:T3)
                n61 = local write "Checkbox"(FALSE ("Checkbox")) -> ()
                n62 = call "SWAY WRITE FGV.vi"("Enum - Menu"=Sway_Write_enum."WRITE", "error in (no error)"=w50, "main ref"=w52) -> ()  [unwired: 8 in, 1 out]
              }
              frame "TEST INCREMENT" {
                n63 = Unbundle By Name(w107) -> ("Motion Module.StepTable For Speed"=w124:refnum<vi>)
                n64 = property class="Tbl (strict)"(reference=w124) -> (reference out=w122:refnum<vi>, error out=w123:errorcluster, "Value"=w121:string[][])  [unwired: 1 in]
                n65 = local read "Time Index"() -> (w142:i32)
                n66 = Close Reference(reference=w122, error in (no error)=w123) -> ()  [unwired: 1 out]
                n67 = Index Array(array=w121, index (row)=w142) -> (element=w137:string[])  [unwired: 1 in]
                n68 = Index Array(array=w137, index #1=1 ("index"), index #2=2 ("index")) -> (element #1=w136:string, element #2=w133:string)
                n69 = Decimal String To Number(string=w136) -> (number=w141:i32)  [unwired: 2 in, 1 out]
                n70 = Unbundle By Name(w107) -> ("Main Screen.Start Test Temp"=w113:refnum<vi>)
                n71 = Unbundle By Name(w107) -> ("Main Screen.STOP"=w118:refnum<vi>)
                n72 = call "ELAPSED TIMER VI FOR STEP SPEED.vi"("TARGET"=w141, "RESET"=FALSE, "PAUSE"=FALSE) -> ("ELAPSED INDICATION"=w135:bool, "ELAPSED TIMER"=→"ELAPSED TIMER":dbl)  [unwired: 6 in, 1 out]
                n73 = property class="Bool (strict)"(reference=w113) -> (reference out=w111:refnum<vi>, error out=w112:errorcluster, "Value"=w114:bool)  [unwired: 1 in]
                n74 = Fract/Exp String To Number(string=w133) -> (number=w126:dbl)  [unwired: 3 in, 1 out]
                n75 = property class="Bool (strict)"(reference=w118) -> (reference out=w120:refnum<vi>, error out=w119:errorcluster, "Value"=w117:bool)  [unwired: 1 in]
                n76 = case shown="False" w135 {
                  tunnel: w126 -> [w144 _]
                  tunnel: w107 -> [w145 _]
                  frame False {
                    n77 = case shown="True" "Checkbox" {
                      selector: "Checkbox" -> [_ w156]
                      tunnel: w145 -> [_ w148]
                      tunnel: w144 -> [_ w147]
                      frame False {
                      }
                      frame True {
                        n78 = Unbundle By Name(w148) -> ("Main Screen.Set Speed"=w160:refnum<vi>)
                        n79 = Not(x=w156) -> (.not. x?=w155:bool)
                        n80 = local write "Checkbox"(w155) -> ()
                        n81 = property class="DigNum (strict)"(reference=w160, "Value"=w147) -> (reference out=w158:refnum<vi>, error out=w159:errorcluster)  [unwired: 1 in]
                        n82 = Bundle By Name(cluster=T4 {"Sequence ID"=0, "Mode Command"=0, "Distance"=0.0, "SPEED"=0.0, "Reserved"=0.0, "SPARE 1"=0, "SPARE 2"=0, "SPARE 3"=0, "SPARE 4"=0, "SPARE 5"=0, "SPARE 6"=0, "SPARE 7"=0, "SPARE 8"=0, "SPARE 9"=0, "SPARE 10"=0, "SPARE 11"=0, "SPARE 12"=0, "SPARE 13"=0, "SPARE 14"=0, "SPARE 15"=0, "SPARE 16"=0, "SPARE 17"=0} ("Value"), "Mode Command"=u8 3, "Distance"=w147) -> (w150:T4)
                        n83 = Unbundle By Name(w148) -> ("SWAY.UPLINK SWAY"=w152:refnum<vi>)
                        n84 = Close Reference(reference=w158, error in (no error)=w159) -> ()  [unwired: 1 out]
                        n85 = property on="Property Node" class="Clust (strict)"(reference=w152, "Value"=w150) -> (reference out=w154:refnum<vi>, error out=w153:errorcluster)  [unwired: 1 in]
                        n86 = Close Reference(reference=w154, error in (no error)=w153) -> (error out=w146:errorcluster)
                        n87 = call "SWAY WRITE FGV.vi"("Enum - Menu"=Sway_Write_enum."WRITE", "error in (no error)"=w146, "main ref"=w148) -> ()  [unwired: 8 in, 1 out]
                      }
                    }
                  }
                  frame True {
                    n88 = local read "Time Index"() -> (w165:i32)
                    n89 = Increment(x=w165) -> (x+1=w164:i32)
                    n90 = local write "Time Index"(w164) -> ()
                    n91 = local write "Checkbox"(TRUE ("Checkbox")) -> ()
                    n92 = call "ELAPSED TIMER VI FOR STEP SPEED.vi"("RESET"=TRUE, "PAUSE"=TRUE) -> ()  [unwired: 7 in, 3 out]
                  }
                }
                n93 = Close Reference(reference=w111, error in (no error)=w112) -> ()  [unwired: 1 out]
                n94 = Close Reference(reference=w120, error in (no error)=w119) -> ()  [unwired: 1 out]
                n95 = Equal?(x=w114, y=FALSE) -> (x = y?=w109:bool)
                n96 = Equal?(x=w117, y=TRUE) -> (x = y?=w110:bool)
                n97 = And(x=w110, y=w109) -> (x .and. y?=w108:bool)
                n98 = local read "Time Index"() -> (w131:i32)
                n99 = local read "Test Size"() -> (w130:i32)
                n100 = Greater Or Equal?(x=w131, y=w130) -> (x >= y?=w129:bool)
                n101 = Or(x=w129, y=w108) -> (x .or. y?=w128:bool)
                n102 = Select(t=STEP_SPEED_SEQUENCE_ENUM."TEST STOP", s=w128, f=STEP_SPEED_SEQUENCE_ENUM."TEST INCREMENT") -> (s? t:f=w127:T3)
              }
              frame "TEST STOP" {
                n103 = Bundle By Name(cluster=T4 {"Sequence ID"=0, "Mode Command"=0, "Distance"=0.0, "SPEED"=0.0, "Reserved"=0.0, "SPARE 1"=0, "SPARE 2"=0, "SPARE 3"=0, "SPARE 4"=0, "SPARE 5"=0, "SPARE 6"=0, "SPARE 7"=0, "SPARE 8"=0, "SPARE 9"=0, "SPARE 10"=0, "SPARE 11"=0, "SPARE 12"=0, "SPARE 13"=0, "SPARE 14"=0, "SPARE 15"=0, "SPARE 16"=0, "SPARE 17"=0} ("Value"), "Mode Command"=u8 5, "Distance"=sgl 0.0, "SPEED"=sgl 10000.0) -> (w175:T4)
                n104 = Unbundle By Name(w166) -> ("Heave AND Surge.UPLINK HEAVE"=w168:refnum<vi>)
                n105 = property on="Property Node" class="Clust (strict)"(reference=w168, "Value"=w175) -> (reference out=w174:refnum<vi>, error out=w173:errorcluster)  [unwired: 1 in]
                n106 = Unbundle By Name(w166) -> ("Main Screen.Start Test"=w182:refnum<vi>)
                n107 = Unbundle By Name(w166) -> ("Main Screen.STOP"=w193:refnum<vi>)
                n108 = Unbundle By Name(w166) -> ("Main Screen.Start Test Temp"=w192:refnum<vi>)
                n109 = Unbundle By Name(w166) -> ("Main Screen.Load En"=w184:refnum<vi>)
                n110 = Close Reference(reference=w174, error in (no error)=w173) -> (error out=w167:errorcluster)
                n111 = property class="Bool (strict)"(reference=w193, "Value"=FALSE, "Visible"=TRUE) -> (reference out=w195:refnum<vi>, error out=w194:errorcluster)  [unwired: 1 in]
                n112 = property class="Bool (strict)"(reference=w192, "Value"=FALSE) -> (reference out=w190:refnum<vi>, error out=w191:errorcluster)  [unwired: 1 in]
                n113 = property class="Bool (strict)"(reference=w184, "Value"=FALSE) -> (reference out=w186:refnum<vi>, error out=w185:errorcluster)  [unwired: 1 in]
                n114 = property class="Bool (strict)"(reference=w182, "Value"=FALSE, "Visible"=TRUE) -> (reference out=w180:refnum<vi>, error out=w181:errorcluster)  [unwired: 1 in]
                n115 = call "SWAY WRITE FGV.vi"("Enum - Menu"=Sway_Write_enum."WRITE", "error in (no error)"=w167, "main ref"=w166) -> ()  [unwired: 8 in, 1 out]
                n116 = Close Reference(reference=w195, error in (no error)=w194) -> ()  [unwired: 1 out]
                n117 = Close Reference(reference=w190, error in (no error)=w191) -> ()  [unwired: 1 out]
                n118 = Close Reference(reference=w186, error in (no error)=w185) -> ()  [unwired: 1 out]
                n119 = Close Reference(reference=w180, error in (no error)=w181) -> ()  [unwired: 1 out]
              }
            }
            n120 = Wait (ms)(milliseconds to wait=u32 300) -> ()  [unwired: 1 out]
          }
        }
      }
    }
    frame Error {
    }
  }
  "error out" <- w1
